vi "Application Data Directory1.vi"(1 "Relative path (.)":path=path "") -> (0 "Application Directory (+ Relative)":path)   [LabVIEW 2015]
doc: "Returns the LV App directory + Relative path."
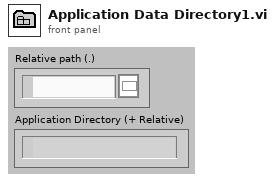
[diagram p1: front panel]
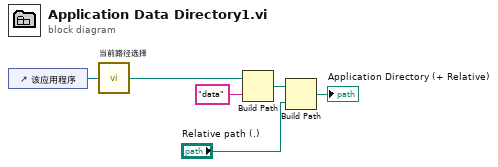
[diagram p0: block diagram]
diagram:
  n1 = control-ref of="该应用程序"() -> (w1:refnum<vi>)
  n2 = call "当前路径选择.vi"("本应用程序"=w1) -> ("当前路径"=w2:path)
  n3 = Build Path(base path=w2, name or relative path="data" ("名称或相对路径")) -> (appended path=w4:path)
  n4 = Build Path(base path=w4, name or relative path="Relative path (.)") -> (appended path=→"Application Directory (+ Relative)":path)
